vi "8-Byte-Array-to-Real-Array.vi"(11 "Data":u8[](array[numeric])=[62, 65, 137, 55, 75, 198, 167, 244, 57, 68, 184, 47, 160, 155, 90, 88] format="%08b") -> (3 "Array of Values":dbl[](array[numeric]))   [LabVIEW 2019]
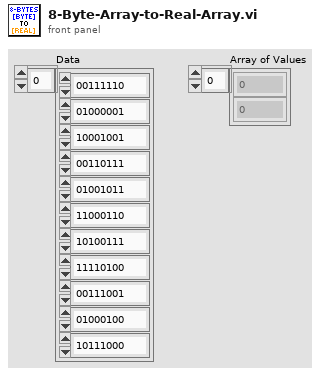
[diagram p1: front panel]
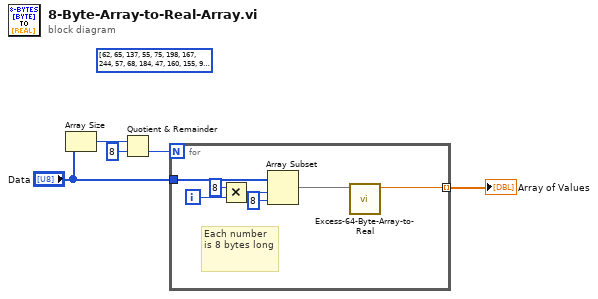
[diagram p0: block diagram]
diagram:
  (unwired) u8[] [62, 65, 137, 55, 75, 198, 167, 244, 57, 68, 184, 47, 160, 155, 90, 88] ("Data")
  n1 = Array Size(array="Data") -> (size(s)=w1:i32)
  n2 = Quotient & Remainder(x=w1, y=8) -> (floor(x/y)=w3:i32)  [unwired: 1 out]
  n3 = for {
    N: w3 -> [_]
    tunnel: [w12] -> w2 mode=indexing
    tunnel: "Data" -> [w11]
    i -> [w8]
    # "Each number is 8 bytes long"
    n4 = Multiply(x=8, y=w8) -> (x*y=w10:i32)
    n5 = Array Subset(array=w11, index=w10, length=8) -> (w6:u8[])
    n6 = call "Excess-64-Byte-Array-to-Real.vi"("Byte array (4 or 8 bytes)"=w6) -> ("Real Number"=w12:dbl)  [unwired: 10 in]
  }
  "Array of Values" <- w2
